vi "ClusterToArray.vi"(8 "error in (no error)":errorcluster caption="Error in (no error)", 11 "Cluster":variant) -> (0 "error out":errorcluster, 3 "Array":variant[](array[variant]))   [LabVIEW 2017]
doc: "Converts a cluster into an array, taking the element type from the cluster's type information so it works for any cluster."
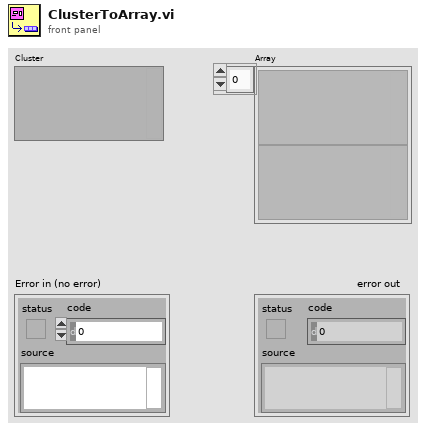
[diagram p1: front panel]
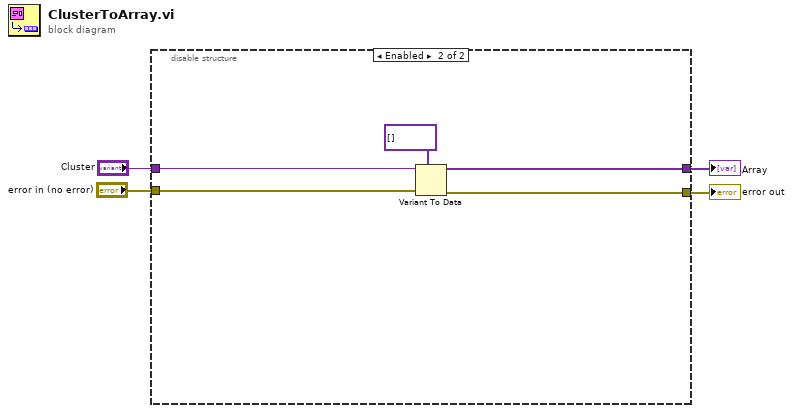
[diagram p0: block diagram]
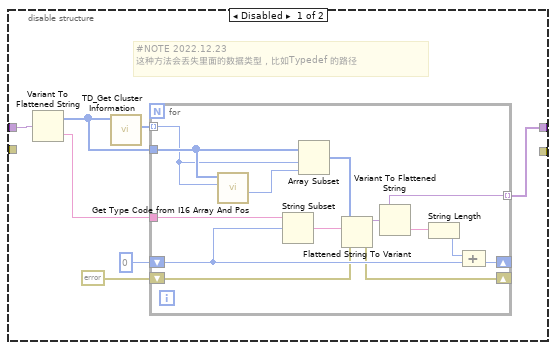
[diagram p2: hidden frame]
diagram:
  n1 = disable-structure shown="Enabled" {
    disable-tunnel: "Cluster" -> [w11 w28]
    disable-tunnel: [w10 w29] -> w3
    disable-tunnel: "error in (no error)" -> [_ w26]
    disable-tunnel: [_ w25] -> w1
    frame Disabled {
      # "#NOTE 2022.12.23\n这种方法会丢失里面的数据类型，比如Typedef 的路径"
      n2 = Variant To Flattened String(Variant=w11) -> (data string=w9:string, 1:w7:i16[])
      n3 = call <vilib>:"TD_Get Cluster Information.vi"("Type descriptor"=w7) -> ("Contained TD Offsets"=w6:i32[])  [unwired: 9 in, 1 out]
      n4 = for {
        tunnel: w7 -> [w15]
        shift-right: [w19] -> _
        shift-left: 0 -> [w20]
        tunnel: w9 -> [w24]
        tunnel: [w18] -> w10 mode=indexing
        shift-right: [w16] -> _
        shift-left: errorcluster {"status"=FALSE, "code"=0, "source"=""} ("error out") -> [w17]
        tunnel: w6 -> [w13] mode=indexing
        n5 = call <vilib>:"Get Type Code from I16 Array And Pos.vi"("Pos in Type Descriptor (0)"=w13, "Type descriptor"=w15) -> ("Size (Words)"=w14:i32)  [unwired: 7 in, 2 out]
        n6 = String Subset(string=w24, offset (0)=w20) -> (substring=w23:string)  [unwired: 1 in]
        n7 = Array Subset(array=w15, index=w13, length=w14) -> (w12:i16[])
        n8 = Flattened String To Variant(4:w17, 6:w23, 7:w12) -> (0:w16:errorcluster, 3:w18:variant)
        n9 = Variant To Flattened String(Variant=w18) -> (data string=w22:string)  [unwired: 1 out]
        n10 = String Length(string=w22) -> (length=w21:i32)
        n11 = Compound Arithmetic op=ADD(w21, w20) -> (w19:i32)
      }
    }
    frame Enabled {
      n12 = Variant To Data(error in=w26, type=variant[] [] ("Array"), Variant=w28) -> (data=w29:variant[], error out=w25:errorcluster)
    }
  }
  "Array" <- w3
  "error out" <- w1
